vi "createClassHierarchyLUT.vi"(8 "error in (no error)":errorcluster, 9 "allClassNames":string[](array[string]), 10 "entireHierarchy":string[][](array[string])) -> (0 "error out":errorcluster, 2 "classHierarchyLUT":map{string, string[]}(c390))   [LabVIEW 2020, in "JKI JSON Object Serialization.lvlib" / "OOP_Utility.lvlib" / "Reflection.lvclass"]
doc: "GCraftsman JSON Object Serialization Toolkit\nwww.GCraftsman.com\nCopyright (c) 2017, GCraftsman"
uses:
  Reflection.lvclass
  Reflection.lvclass/Reflection.ctl
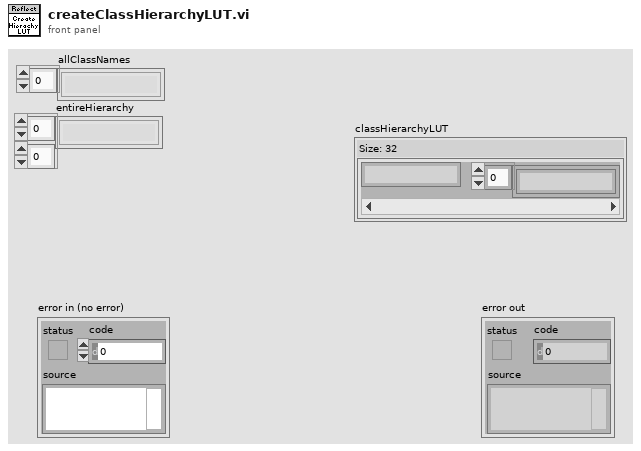
[diagram p1: front panel]
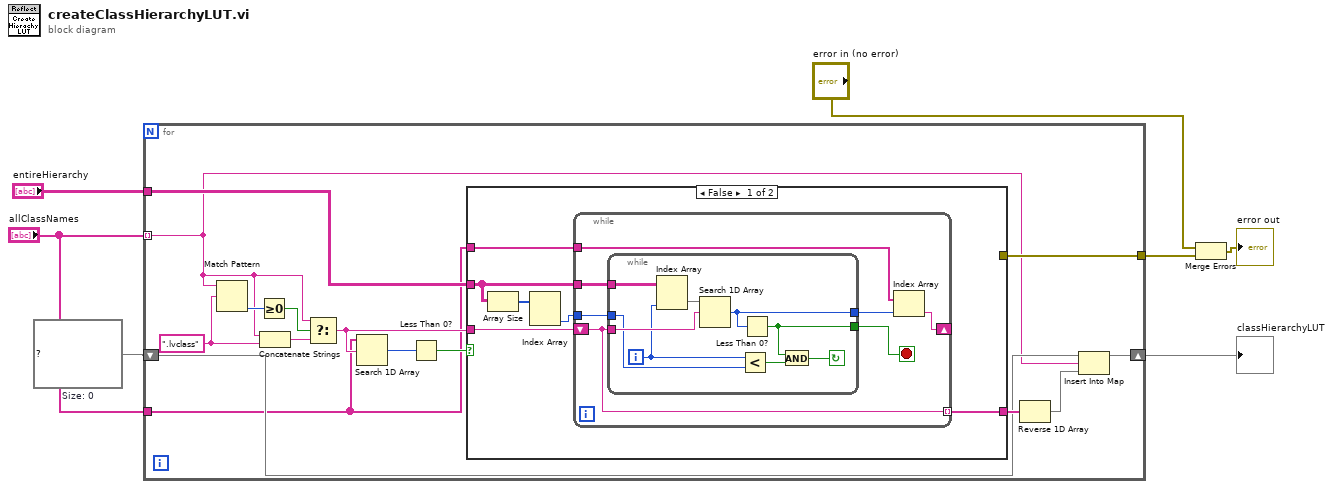
[diagram p0: block diagram]
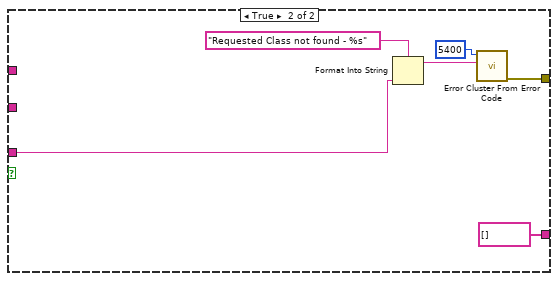
[diagram p2: hidden frame]
diagram:
  w1 = map{string, string[]} {}  # Size: 0
  n1 = for {
    tunnel: [w22] -> w7
    tunnel: "entireHierarchy" -> [w13]
    tunnel: "allClassNames" -> [w11] mode=indexing
    shift-right: [w9] -> w3
    shift-left: w1 -> [w12]
    tunnel: "allClassNames" -> [w8]
    w16 = ".lvclass" ("regular expression")
    n2 = Match Pattern(string=w11, regular expression=w16) -> (offset past match=w18:i32)  [unwired: 1 in, 3 out]
    n3 = Greater Or Equal To 0?(x=w18) -> (x >= 0?=w17:bool)
    n4 = Concatenate Strings(w11, w16) -> (w15:string)
    n5 = Select(t=w11, s=w17, f=w15) -> (s? t:f=w14:string)
    n6 = Search 1D Array(1D array=w8, element=w14) -> (index of element=w21:i32)  [unwired: 1 in]
    n7 = Less Than 0?(x=w21) -> (x < 0?=w20:bool)
    n8 = case shown="False" w20 {
      tunnel: w14 -> [w26 w49]
      tunnel: [_ w47] -> w22
      tunnel: w13 -> [w24 _]
      tunnel: [w25 string[] []] -> w19
      tunnel: w8 -> [w23 _]
      frame False {
        n9 = Array Size(array=w24) -> (size(s)=w27:i32[])
        n10 = Index Array(array=w27) -> (element #2=w28:i32)  [unwired: 2 in, 1 out]
        n11 = while {
          tunnel: w24 -> [w35]
          shift-right: [w31] -> _
          shift-left: w26 -> [w30]
          tunnel: w23 -> [w32]
          tunnel: [w30] -> w25 mode=indexing
          tunnel: w28 -> [w29]
          stop <- w33 stop-if-true
          n12 = while {
            tunnel: w35 -> [w42]
            tunnel: w30 -> [w44]
            tunnel: [w43] -> w34
            tunnel: [w38] -> w33
            tunnel: w29 -> [w39]
            i -> [w40]
            stop <- w36 continue-if-true
            n13 = Index Array(array=w42, index (col)=w40) -> (element=w41:string[])  [unwired: 1 in]
            n14 = Search 1D Array(1D array=w41, element=w44) -> (index of element=w43:i32)  [unwired: 1 in]
            n15 = Less?(x=w40, y=w39) -> (x < y?=w37:bool)
            n16 = Less Than 0?(x=w43) -> (x < 0?=w38:bool)
            n17 = And(x=w38, y=w37) -> (x .and. y?=w36:bool)
          }
          n18 = Index Array(array=w32, index=w34) -> (element=w31:string)
        }
      }
      frame True {
        n19 = Format Into String(format string="Requested Class not found - %s" ("message"), w49) -> (resulting string=w48:string)  [unwired: 2 in, 1 out]
        n20 = call <vilib>:"Error Cluster From Error Code.vi"("error message (\"\")"=w48, "error code (0)"=5400) -> ("error out"=w47:errorcluster)  [unwired: 7 in]
      }
    }
    n21 = Reverse 1D Array(array=w19) -> (reversed array=w10:string[])
    n22 = Insert Into Map(map in=w12, key=w11, value=w10) -> (map out=w9:map{string, string[]})  [unwired: 2 out]
  }
  "classHierarchyLUT" <- w3
  n23 = Merge Errors("error in (no error)", w7) -> (→"error out":errorcluster)
